vi "HaskellActive.vi"() -> ()   [LabVIEW 2013]
panel:
  out "HaskellActive":bool
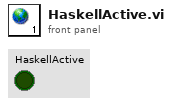
[diagram p1: front panel]
diagram:
